vi "gyro.vi"() -> (6 "Angle":dbl, 7 "Full Angle":dbl, 8 "Angular Rate":dbl)   [LabVIEW 2014]
uses:
  <vilib>/Rock Robotics/Network Tables/NT Read Numeric Array.vi
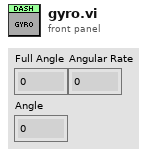
[diagram p1: front panel]
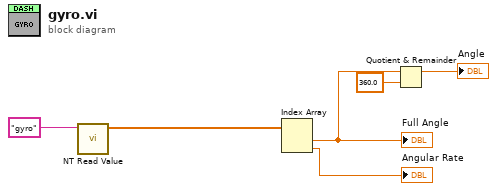
[diagram p0: block diagram]
diagram:
  n1 = call-poly <vilib>:"NT Read Value.vi"("Name"="gyro") -> ("Numeric Array"=w6:dbl[])  [unwired: 9 in, 1 out]
  n2 = Index Array(array=w6) -> (element #1=w4:dbl, element #2=→"Angular Rate":dbl)  [unwired: 2 in]
  "Full Angle" <- w4
  n3 = Quotient & Remainder(x=w4, y=360.0) -> (x-y*floor(x/y)=→"Angle":dbl)  [unwired: 1 out]
